vi "sv_Triangle Wave with Duty Cycle.vi"(6 "duty cycle [%]":dbl=50.0 format="%0.2f", 8 "phase in [deg]":dbl format="%0.2f", 9 "normalized frequency (f/Fs)":dbl=0.0078125 format="%0.4e", 10 "amplitude":dbl=1.0 format="%0.2f", 11 "samples":i32=128) -> (0 "phase out":dbl format="%0.2e", 3 "triangle wave":dbl[](array[numeric]))   [LabVIEW 2017, in "SV Triangle.lvclass"]
uses:
  <vilib>/addons/_NISVFA/_Generation/Signal Generation/SV Triangle/SV Triangle.lvclass
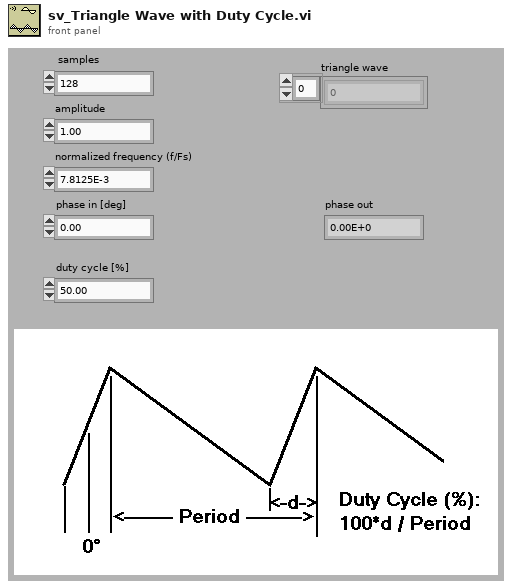
[diagram p1: front panel]
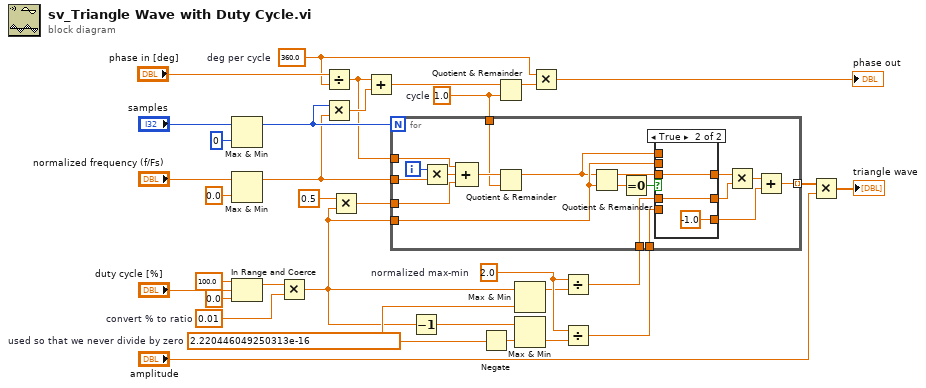
[diagram p0: block diagram]
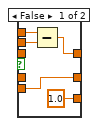
[diagram p2: hidden frame]
diagram:
  w7 = 1.0  # cycle
  w10 = 2.220446049250313e-16  # used so that we never divide by zero
  w28 = 2.0  # normalized max-min
  w6 = 360.0  # deg per cycle
  w30 = 0.01  # convert % to ratio
  n1 = Max & Min(x="samples", y=0 ("lower limit")) -> (max(x,y)=w23:i32)  [unwired: 1 out]
  n2 = Max & Min(x="normalized frequency (f/Fs)", y=0.0 ("lower limit")) -> (max(x,y)=w15:dbl)  [unwired: 1 out]
  n3 = In Range and Coerce(upper limit=100.0, x="duty cycle [%]", lower limit=0.0) -> (coerced(x)=w19:dbl)  [unwired: 1 out]
  n4 = Multiply(x=w19, y=w30) -> (x*y=w3:dbl)
  n5 = Divide(x="phase in [deg]", y=w6) -> (x/y=w8:dbl)
  n6 = Multiply(x=w23, y=w15) -> (x*y=w25:dbl)
  n7 = Multiply(x=0.5, y=w3) -> (x*y=w1:dbl)
  n8 = Add(x=w8, y=w25) -> (x+y=w22:dbl)
  n9 = Decrement(x=w3) -> (x-1=w13:dbl)
  n10 = Negate(x=w10) -> (-x=w11:dbl)
  n11 = Quotient & Remainder(x=w22, y=w7) -> (x-y*floor(x/y)=w5:dbl)  [unwired: 1 out]
  n12 = Max & Min(x=w3, y=w10) -> (max(x,y)=w14:dbl)  [unwired: 1 out]
  n13 = Max & Min(x=w13, y=w11) -> (min(x,y)=w12:dbl)  [unwired: 1 out]
  n14 = Multiply(x=w6, y=w5) -> (x*y=→"phase out":dbl)
  n15 = Divide(x=w28, y=w14) -> (x/y=w27:dbl)
  n16 = Divide(x=w28, y=w12) -> (x/y=w26:dbl)
  n17 = for {
    N: w23 -> [_]
    tunnel: w3 -> [w42]
    tunnel: [w43] -> w29 mode=indexing
    tunnel: w27 -> [w49]
    tunnel: w26 -> [w48]
    tunnel: w15 -> [w40]
    tunnel: w1 -> [w35]
    tunnel: w8 -> [w37]
    tunnel: w7 -> [w34]
    i -> [w41]
    n18 = Multiply(x=w41, y=w40) -> (x*y=w38:dbl)
    n19 = Compound Arithmetic op=ADD(w37, w38, w35) -> (w36:dbl)
    n20 = Quotient & Remainder(x=w36, y=w34) -> (x-y*floor(x/y)=w39:dbl)  [unwired: 1 out]
    n21 = Quotient & Remainder(x=w39, y=w42) -> (x-y*floor(x/y)=w50:dbl, floor(x/y)=w52:dbl)
    n22 = Equal To 0?(x=w52) -> (x = 0?=w51:bool)
    n23 = case shown="True" w51 {
      tunnel: w50 -> [_ w60]
      tunnel: w49 -> [_ w59]
      tunnel: w48 -> [w53 _]
      tunnel: [w54 w60] -> w47
      tunnel: [w53 w59] -> w46
      tunnel: [1.0 -1.0] -> w44
      tunnel: w39 -> [w56 _]
      tunnel: w42 -> [w55 _]
      frame False {
        n24 = Subtract(x=w56, y=w55) -> (x-y=w54:dbl)
      }
      frame True {
      }
    }
    n25 = Multiply(x=w47, y=w46) -> (x*y=w45:dbl)
    n26 = Add(x=w45, y=w44) -> (x+y=w43:dbl)
  }
  n27 = Multiply(x=w29, y="amplitude") -> (x*y=→"triangle wave":dbl[])
